vi "Upload File.vi"(6 "Chunk size (kB)":i32=5120 min=5120, 8 "error in (no error)":errorcluster, 9 "Object Path (including file name)":string, 10 "file to upload":path, 11 "Data.S3":refnum<class "LV-Data.S3.lvclass">) -> (0 "error out":errorcluster, 3 "Data.S3":refnum<class "LV-Data.S3.lvclass">)   [LabVIEW 2016, in "LV-Data.S3.lvclass"]
uses:
  LV-Data.S3.lvclass
  LV-Data.S3.lvclass/LV-Data.S3.ctl
  <vilib>/AWS Toolkit/S3/Bucket/Bucket.lvclass
panel:
  # "* an object path includes the name of the file, and does not include\nthe bucket name. e.g:\nPPMS2/SA03008N.20190801/031_sideGateSweep.tdms"
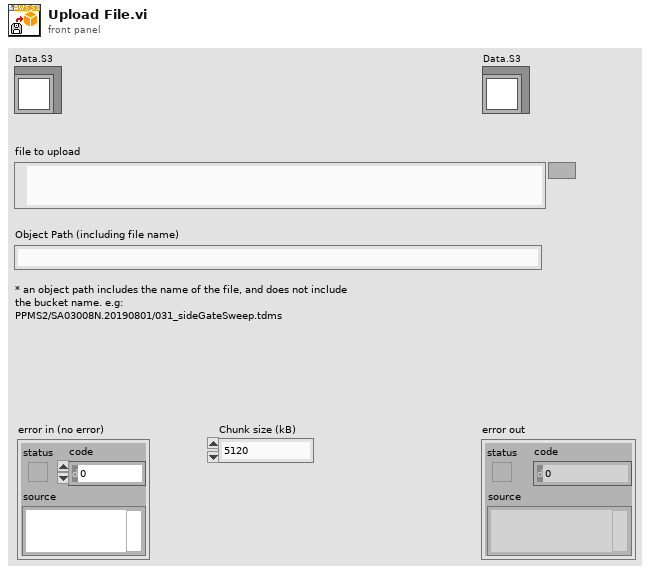
[diagram p1: front panel]
types:
  T1 = typedef "NI_AWS_Core.lvlib/HTTP Request.lvclass/AWS Credentials.ctl" = cluster{"Access Key":string, "Secret Key":string}
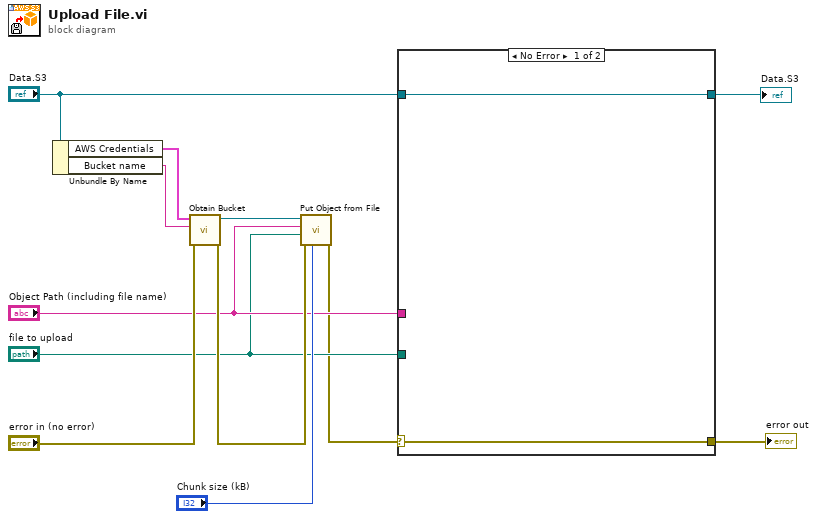
[diagram p0: block diagram]
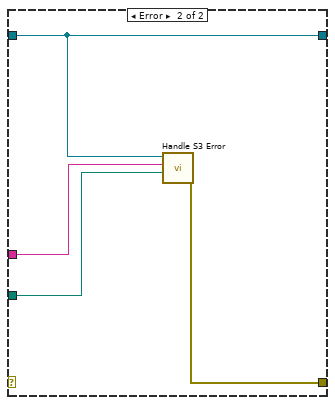
[diagram p2: hidden frame]
diagram:
  n1 = Unbundle By Name("Data.S3") -> ("AWS Credentials"=w8:T1, "Bucket name"=w7:string)
  n2 = call <vilib>:"Obtain Bucket.vi"("error in (no error)"="error in (no error)", "Bucket name"=w7, "AWS Credentials"=w8) -> ("error out"=w11:errorcluster, "Bucket"=w10:refnum<class "Bucket.lvclass">)  [unwired: 7 in]
  n3 = call <vilib>:"Put Object from File.vi"("Chunk size (kB)"="Chunk size (kB)", "error in (no error)"=w11, "File"="file to upload", "Object Path"="Object Path (including file name)", "Bucket in"=w10) -> ("error out"=w3:errorcluster)  [unwired: 2 in, 4 out]
  n4 = case shown="No Error" w3 {
    selector: w3 -> [w14 _]
    tunnel: "Data.S3" -> [w13 w15]
    tunnel: "Object Path (including file name)" -> [_ w18]
    tunnel: "file to upload" -> [_ w17]
    tunnel: [w14 w16] -> w2
    tunnel: [w13 w15] -> w1
    frame No Error {
    }
    frame Error {
      n5 = call "Handle S3 Error.vi"("File Path"=w17, "Object Path"=w18, "Data.S3 in"=w15) -> ("error out"=w16:errorcluster)  [unwired: 6 in, 2 out]
    }
  }
  "error out" <- w2
  "Data.S3" <- w1
